vi "Read Lengths.vi"(0 "TDMS In":refnum<k34>, 11 "Error In":errorcluster) -> (4 "TDMS Out":refnum<k34>, 6 "# Inputs":i32, 8 "# Outputs":i32, 10 "# Samples":i64, 15 "Error Out":errorcluster)   [LabVIEW 2015, in "Teaching File.lvlib"]
doc: "Read the # channels and the # samples in Input_Data and Output_Data groups."
uses:
  Teaching File.lvlib
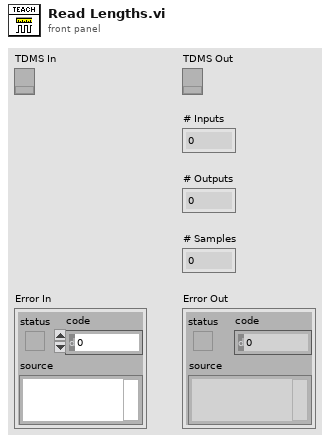
[diagram p1: front panel]
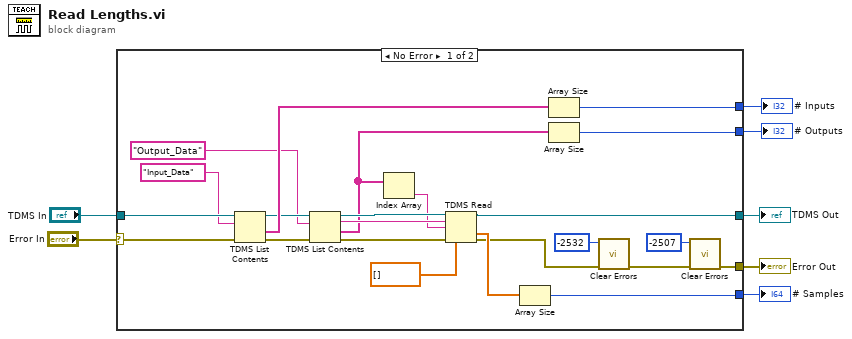
[diagram p0: block diagram]
diagram:
  n1 = case shown="No Error" "Error In" {
    selector: "Error In" -> [w19 w31]
    tunnel: "TDMS In" -> [w30 _]
    tunnel: [w26 _] -> w6
    tunnel: [w24 _] -> w5
    tunnel: [w9 _] -> w4
    tunnel: [w11 _] -> w3
    tunnel: [w20 w31] -> w2
    frame No Error {
      n2 = TDMS List Contents(4:w19, 6:"Input_Data" ("group name"), 7:w30) -> (0:w28:errorcluster, 1:w27:string[], 3:w25:refnum<k34>)  [unwired: 1 out]
      n3 = TDMS List Contents(4:w28, 6:"Output_Data" ("group name"), 7:w25) -> (0:w16:errorcluster, 1:w14:string[], 2:w15:string, 3:w17:refnum<k34>)
      n4 = Index Array(array=w14) -> (element=w13:string)  [unwired: 1 in]
      n5 = TDMS Read(0:w17, 5:w15, 7:w13, 11:w16, 12:dbl[] []) -> (4:w9:refnum<k34>, 10:w10:dbl[], 15:w8:errorcluster)  [unwired: 3 in, 3 out]
      n6 = Array Size(array=w10) -> (size(s)=w11:i32)
      n7 = Array Size(array=w27) -> (size(s)=w26:i32)
      n8 = Array Size(array=w14) -> (size(s)=w24:i32)
      n9 = call <vilib>:"Clear Errors.vi"("error in (no error)"=w8, "specific error code to clear (0: all)"=-2532) -> ("error out"=w22:errorcluster)  [unwired: 4 in, 1 out]
      n10 = call <vilib>:"Clear Errors.vi"("error in (no error)"=w22, "specific error code to clear (0: all)"=-2507) -> ("error out"=w20:errorcluster)  [unwired: 4 in, 1 out]
    }
    frame Error {
    }
  }
  "Error Out" <- w2
  "TDMS Out" <- w4
  "# Inputs" <- w6
  "# Outputs" <- w5
  "# Samples" <- w3
